vi "Initialize.vi"(0 "VISA resource name":refnum<visa-resource-name>, 1 "ID Query (True)":bool=TRUE, 2 "Reset (False)":bool, 3 "error in (no error)":errorcluster, 4 "Serial Link (RS232)":enum16{"RS232", "USB"}(ring)) -> (7 "VISA resource name out":refnum<visa-resource-name>, 10 "error out":errorcluster {"code" format="%.0x"})   [LabVIEW 2020, in "Newport ESP301.lvlib"]
doc: "Establishes communication with the instrument and optionally performs an instrument identification query and/or an instrument reset. It also places the instrument in a default state needed for other instrument driver operations. Therefore, call this VI before calling other instrument driver VIs for this instrument. Generally, you need to call the Initialize VI only once at the beginning of an application."
uses:
  Newport ESP301.lvlib
panel:
  # "(c) 2009 - 2013 Newport Corporation"
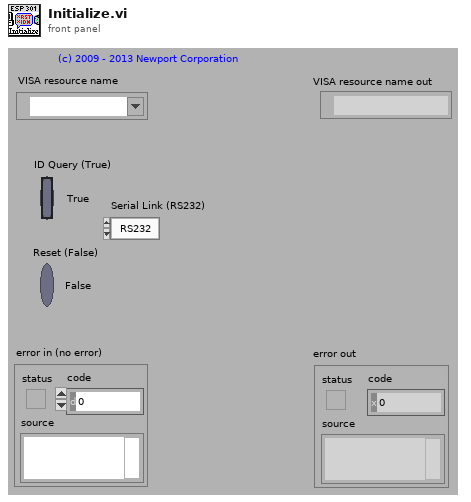
[diagram p1: front panel]
types:
  T1 = cluster{"Baud Rate":u32, "Parity":u16, "Data Bits":u16, "Stop Bits":u16, "Flow Control":u16}
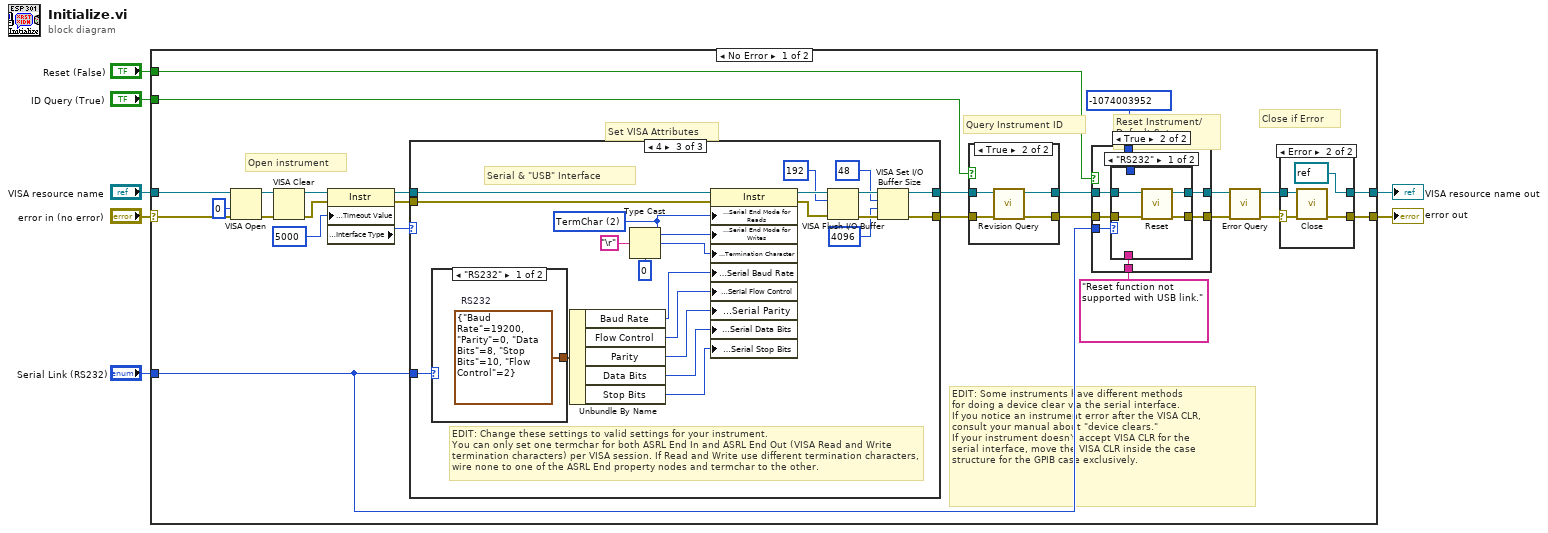
[diagram p0: block diagram]
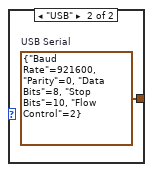
[diagram p5: hidden frame]
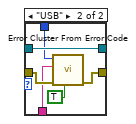
[diagram p7: hidden frame]
diagram:
  n1 = case shown="No Error" "error in (no error)" {
    selector: "error in (no error)" -> [w15 w94]
    tunnel: "ID Query (True)" -> [w31 _]
    tunnel: "Reset (False)" -> [w30 _]
    tunnel: "VISA resource name" -> [w29 w93]
    tunnel: [w11 w93] -> w2
    tunnel: [w13 w94] -> w1
    tunnel: "Serial Link (RS232)" -> [w10 _]
    frame No Error {
      # "EDIT: Some instruments have different methods\nfor doing a device clear via the serial interface.  \nIf you notice an instrument error after the VISA CLR,\nconsult your manual about \"device clears.\"  \nIf your instrument doesn't accept VISA CLR for the\nserial interface, move the VISA CLR inside the case \nstructure for the GPIB case exclusively."
      # "Set VISA Attributes"
      # "Close if Error"
      # "Query Instrument ID"
      # "Reset Instrument/\nDefault Setup"
      # "Open instrument"
      n2 = VISA Open(access mode=u32 0, error in (no error)=w15, VISA resource name=w29) -> (VISA resource name=w22:refnum<visa-resource-name>, error out=w21:errorcluster)  [unwired: 2 out]
      n3 = VISA Clear(VISA resource name=w22, error in (no error)=w21) -> (VISA resource name out=w20:refnum<visa-resource-name>, error out=w19:errorcluster)
      n4 = property class="Instr"(reference=w20, error in=w19, "General Settings:Timeout Value"=u32 5000) -> (reference out=w25:refnum<visa-resource-name>, error out=w24:errorcluster, "Interface Information:Interface Type"=w16:u16)
      n5 = case shown="4" w16 {
        tunnel: [w40 w43 w62] -> w27
        tunnel: [w41 w42 w59] -> w26
        tunnel: w25 -> [w40 w43 w64]
        tunnel: w24 -> [w41 w42 w65]
        tunnel: w10 -> [_ _ w46]
        frame Default {
          # "TCP/IP, and USB Interface"
        }
        frame 1 {
          # "GPIB Interface"
        }
        frame 4 {
          w53 = u16 2 items=["None", "LastBit", "TermChar"] ("Serial Settings:Serial End Mode for Reads")
          # "EDIT: Change these settings to valid settings for your instrument.\nYou can only set one termchar for both ASRL End In and ASRL End Out (VISA Read and Write termination characters) per VISA session. If Read and Write use different termination characters, wire none to one of the ASRL End property nodes and termchar to the other."
          # "Serial & \"USB\" Interface"
          n6 = case shown="\"RS232\"" w46 {
            tunnel: [w66 w67] -> w45
            frame "RS232" {
              w66 = T1 {"Baud Rate"=19200, "Parity"=0, "Data Bits"=8, "Stop Bits"=10, "Flow Control"=2}  # RS232
            }
            frame "USB" {
              w67 = T1 {"Baud Rate"=921600, "Parity"=0, "Data Bits"=8, "Stop Bits"=10, "Flow Control"=2}  # USB Serial
            }
          }
          n7 = Unbundle By Name(w45) -> ("Baud Rate"=w51:u32, "Flow Control"=w48:u16, "Parity"=w49:u16, "Data Bits"=w50:u16, "Stop Bits"=w47:u16)
          n8 = Type Cast(type=u8 0, x="\r") -> (*(type *) &x=w52:u8)
          n9 = property class="Instr"(reference=w64, error in=w65, "Serial Settings:Serial End Mode for Reads"=w53, "Serial Settings:Serial End Mode for Writes"=w53, "Message Based Settings:Termination Character"=w52, "Serial Settings:Serial Baud Rate"=w51, "Serial Settings:Serial Flow Control"=w48, "Serial Settings:Serial Parity"=w49, "Serial Settings:Serial Data Bits"=w50, "Serial Settings:Serial Stop Bits"=w47) -> (reference out=w58:refnum<visa-resource-name>, error out=w61:errorcluster)
          n10 = VISA Flush I/O Buffer(VISA resource name=w58, mask (16)=u16 192, error in (no error)=w61) -> (VISA resource name out=w63:refnum<visa-resource-name>, error out=w60:errorcluster)
          n11 = VISA Set I/O Buffer Size(VISA resource name=w63, mask (16)=u16 48, size (4096)=u32 4096 ("size (0)"), error in (no error)=w60) -> (VISA resource name out=w62:refnum<visa-resource-name>, error out=w59:errorcluster)
        }
      }
      n12 = case shown="True" w31 {
        tunnel: [w87 w89] -> w32
        tunnel: [w88 w91] -> w33
        tunnel: w27 -> [w88 w92]
        tunnel: w26 -> [w87 w90]
        frame False {
        }
        frame True {
          n13 = call "Revision Query.vi"("error in (no error)"=w90, "VISA resource name"=w92) -> ("error out"=w89:errorcluster, "VISA resource name out"=w91:refnum<visa-resource-name>)  [unwired: 8 out]
        }
      }
      n14 = case shown="True" w30 {
        tunnel: w32 -> [w68 w73]
        tunnel: [w68 w76] -> w17
        tunnel: w33 -> [w69 w74]
        tunnel: [w69 w75] -> w18
        tunnel: w10 -> [_ w72]
        tunnel: -1074003952 ("Code") -> [_ w71]
        tunnel: "Reset function not supported with USB link." ("Source (VI Name)") -> [_ w70]
        frame False {
        }
        frame True {
          n15 = case shown="\"RS232\"" w72 {
            tunnel: [w80 w83] -> w76
            tunnel: [w79 w86] -> w75
            tunnel: w74 -> [w78 w86]
            tunnel: w73 -> [w77 w84]
            tunnel: w71 -> [_ w82]
            tunnel: w70 -> [_ w81]
            frame "RS232" {
              n16 = call "Reset.vi"("error in (no error)"=w77, "VISA resource name"=w78) -> ("error out"=w80:errorcluster, "VISA resource name out"=w79:refnum<visa-resource-name>)  [unwired: 4 out]
            }
            frame "USB" {
              n17 = call <vilib>:"Error Cluster From Error Code.vi"("show call chain? (False)"=TRUE, "error in (no error)"=w84, "error message (\"\")"=w81, "error code (0)"=w82) -> ("error out"=w83:errorcluster)  [unwired: 5 out]
            }
          }
        }
      }
      n18 = call "Error Query.vi"("error in (no error)"=w17, "VISA resource name"=w18) -> ("error out"=w14:errorcluster, "VISA resource name out"=w12:refnum<visa-resource-name>)  [unwired: 4 out]
      n19 = case shown="Error" w14 {
        selector: w14 -> [w35 w37]
        tunnel: w12 -> [w34 w38]
        tunnel: [w34 refnum<visa-resource-name> refnum ("VISA resource name out")] -> w11
        tunnel: [w35 w39] -> w13
        frame No Error {
        }
        frame Error {
          n20 = call "Close.vi"("error in (no error)"=w37, "VISA resource name"=w38) -> ("error out"=w39:errorcluster)  [unwired: 9 out]
        }
      }
    }
    frame Error {
    }
  }
  "VISA resource name out" <- w2
  "error out" <- w1
